vi "mxwScript_Cmnd2Str_setStringTableEntries.vi"(8 "error in (no error)":errorcluster, 11 "data":variant) -> (0 "error out":errorcluster, 3 "outputString":string)   [LabVIEW 2017]
uses:
  codeGenAPISupport.llb/cgAPI_mxwScript_StrTbl_StringTableItem.ctl
  codeGenAPISupport.llb/cgAPI_mxwScript_StrTbl_StringTableSelector.ctl
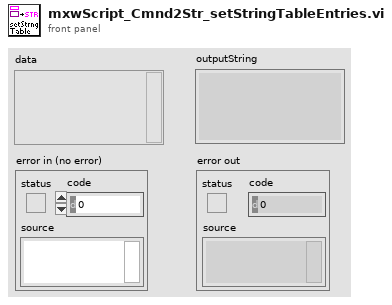
[diagram p1: front panel]
types:
  T1 = typedef "cgAPI_mxwScript_StrTbl_StringTableItem.ctl" = cluster{"stringTableSelection":T2, "tableIndex":i32, "tableString":string}
  T2 = typedef "cgAPI_mxwScript_StrTbl_StringTableSelector.ctl" = enum16{"target", "engine"}
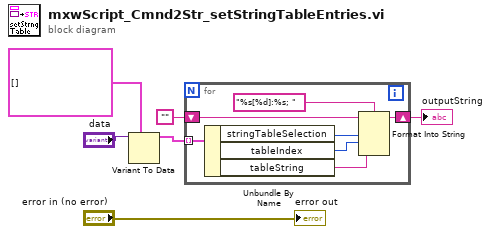
[diagram p0: block diagram]
diagram:
  n1 = Variant To Data(type=T1[] [], Variant="data") -> (data=w3:T1[])  [unwired: 1 in, 1 out]
  n2 = for {
    tunnel: w3 -> [w10] mode=indexing
    shift-right: [w12] -> w1
    shift-left: "" -> [w11]
    n3 = Unbundle By Name(w10) -> ("stringTableSelection"=w9:T2, "tableIndex"=w8:i32, "tableString"=w7:string)
    n4 = Format Into String(format string="%s[%d]:%s; ", initial string=w11, w9, w8, w7) -> (resulting string=w12:string)  [unwired: 1 in, 1 out]
  }
  "outputString" <- w1
  "error out" <- "error in (no error)"
